vi "6733_Write_daqmx.vi"(0 "Arbitrary Waveform\nArray of Channels":T1(array[cluster])=[[{"AC Frequency (kHz)"=40.0, " Initial AC Ampl. (p-p/2)"=0.0, "Final AC Ampl."=0.0, "Initial DC Value"=-1.0, "Final DC Value"=-0.58, "Constant"=179.88, "Gamma AC"=1.0, "String"="Channel 0 A", "Gamma DC"=1.0}, {"AC Frequency (kHz)"=40.0, " Initial AC Ampl. (p-p/2)"=0.0, "Final AC Ampl."=0.0, "Initial DC Value"=-0.58, "Final DC Value"=-0.095, "Constant"=179.88, "Gamma AC"=1.0, "String"="Channel 0 B", "Gamma DC"=1.0}, {"AC Frequency (kHz)"=40.0, " Initial AC Ampl. (p-p/2)"=0.0, "Final AC Ampl."=0.0, "Initial DC Value"=-0.095, "Final DC Value"=-0.03, "Constant"=179.88, "Gamma AC"=1.0, "String"="Channel 0 C", "Gamma DC"=1.0}, {"AC Frequency (kHz)"=0.0, " Initial AC Ampl. (p-p/2)"=0.0, "Final AC Ampl."=0.0, "Initial DC Value"=0.0, "Final DC Value"=0.0, "Constant"=179.88, "Gamma AC"=0.0, "String"="Channel 0 D", "Gamma DC"=1.0}], [{"AC Frequency (kHz)"=10.0, " Initial AC Ampl. (p-p/2)"=5.0, "Final AC Ampl."=0.0, "Initial DC Value"=0.17, "Final DC Value"=0.095, "Constant"=0.25, "Gamma AC"=1.0, "String"="Channel 1 A", "Gamma DC"=1.0}, {"AC Frequency (kHz)"=10.0, " Initial AC Ampl. (p-p/2)"=5.0, "Final AC Ampl."=0.0, "Initial DC Value"=0.095, "Final DC Value"=0.009, "Constant"=0.25, "Gamma AC"=1.0, "String"="Channel 1 B", "Gamma DC"=1.0}, {"AC Frequency (kHz)"=10.0, " Initial AC Ampl. (p-p/2)"=0.0, "Final AC Ampl."=0.0, "Initial DC Value"=0.009, "Final DC Value"=0.001, "Constant"=0.25, "Gamma AC"=1.0, "String"="Channel 1 C", "Gamma DC"=1.0}, {"AC Frequency (kHz)"=0.0, " Initial AC Ampl. (p-p/2)"=0.0, "Final AC Ampl."=0.0, "Initial DC Value"=0.001, "Final DC Value"=0.001, "Constant"=0.25, "Gamma AC"=0.0, "String"="Channel 1 D", "Gamma DC"=1.0}], [{"AC Frequency (kHz)"=10.0, " Initial AC Ampl. (p-p/2)"=0.0, "Final AC Ampl."=0.0, "Initial DC Value"=0.006, "Final DC Value"=0.01, "Constant"=0.0, "Gamma AC"=1.0, "String"="Channel 2 A", "Gamma DC"=1.0}, {"AC Frequency (kHz)"=10.0, " Initial AC Ampl. (p-p/2)"=0.0, "Final AC Ampl."=0.0, "Initial DC Value"=0.01, "Final DC Value"=0.04, "Constant"=0.0, "Gamma AC"=1.0, "String"="Channel 2 B", "Gamma DC"=1.0}, {"AC Frequency (kHz)"=10.0, " Initial AC Ampl. (p-p/2)"=0.0, "Final AC Ampl."=0.0, "Initial DC Value"=0.04, "Final DC Value"=0.04, "Constant"=0.0, "Gamma AC"=1.0, "String"="Channel 2 C", "Gamma DC"=1.0}, {"AC Frequency (kHz)"=0.0, " Initial AC Ampl. (p-p/2)"=0.0, "Final AC Ampl."=0.0, "Initial DC Value"=0.04, "Final DC Value"=0.04, "Constant"=0.0, "Gamma AC"=0.0, "String"="Channel 2 D", "Gamma DC"=1.0}], [{"AC Frequency (kHz)"=10.0, " Initial AC Ampl. (p-p/2)"=0.0, "Final AC Ampl."=0.0, "Initial DC Value"=10.0, "Final DC Value"=10.0, "Constant"=199.2, "Gamma AC"=1.0, "String"="Channel 3 A", "Gamma DC"=1.0}, {"AC Frequency (kHz)"=10.0, " Initial AC Ampl. (p-p/2)"=0.0, "Final AC Ampl."=0.0, "Initial DC Value"=10.0, "Final DC Value"=1.0, "Constant"=199.2, "Gamma AC"=1.0, "String"="Channel 3 B", "Gamma DC"=1.0}, {"AC Frequency (kHz)"=10.0, " Initial AC Ampl. (p-p/2)"=0.0, "Final AC Ampl."=0.0, "Initial DC Value"=1.0, "Final DC Value"=0.9, "Constant"=199.2, "Gamma AC"=1.0, "String"="Channel 3 C", "Gamma DC"=1.0}, {"AC Frequency (kHz)"=0.0, " Initial AC Ampl. (p-p/2)"=0.0, "Final AC Ampl."=0.0, "Initial DC Value"=5.0, "Final DC Value"=5.0, "Constant"=199.2, "Gamma AC"=1.0, "String"="Channel 3 D", "Gamma DC"=1.0}], [{"AC Frequency (kHz)"=10.0, " Initial AC Ampl. (p-p/2)"=0.0, "Final AC Ampl."=0.0, "Initial DC Value"=2.445, "Final DC Value"=2.445, "Constant"=0.0, "Gamma AC"=1.0, "String"="Channel 4 A", "Gamma DC"=1.0}, {"AC Frequency (kHz)"=10.0, " Initial AC Ampl. (p-p/2)"=0.0, "Final AC Ampl."=0.0, "Initial DC Value"=2.445, "Final DC Value"=2.432, "Constant"=0.0, "Gamma AC"=1.0, "String"="Channel 4 B", "Gamma DC"=1.0}, {"AC Frequency (kHz)"=10.0, " Initial AC Ampl. (p-p/2)"=0.0, "Final AC Ampl."=0.0, "Initial DC Value"=2.432, "Final DC Value"=2.432, "Constant"=0.0, "Gamma AC"=1.0, "String"="Channel 4 C", "Gamma DC"=1.0}, {"AC Frequency (kHz)"=0.0, " Initial AC Ampl. (p-p/2)"=0.0, "Final AC Ampl."=0.0, "Initial DC Value"=2.432, "Final DC Value"=2.432, "Constant"=0.0, "Gamma AC"=0.0, "String"="Channel 4 D", "Gamma DC"=1.0}], [{"AC Frequency (kHz)"=10.0, " Initial AC Ampl. (p-p/2)"=0.0, "Final AC Ampl."=0.0, "Initial DC Value"=6.46, "Final DC Value"=6.46, "Constant"=0.0, "Gamma AC"=1.0, "String"="Channel 5 A", "Gamma DC"=1.0}, {"AC Frequency (kHz)"=10.0, " Initial AC Ampl. (p-p/2)"=0.0, "Final AC Ampl."=0.0, "Initial DC Value"=6.46, "Final DC Value"=6.46, "Constant"=0.0, "Gamma AC"=1.0, "String"="Channel 5 B", "Gamma DC"=1.0}, {"AC Frequency (kHz)"=10.0, " Initial AC Ampl. (p-p/2)"=0.0, "Final AC Ampl."=0.0, "Initial DC Value"=6.46, "Final DC Value"=6.46, "Constant"=0.0, "Gamma AC"=1.0, "String"="Channel 5 C", "Gamma DC"=1.0}, {"AC Frequency (kHz)"=0.0, " Initial AC Ampl. (p-p/2)"=0.0, "Final AC Ampl."=0.0, "Initial DC Value"=6.46, "Final DC Value"=6.46, "Constant"=0.0, "Gamma AC"=0.0, "String"="Channel 5 D", "Gamma DC"=1.0}], [{"AC Frequency (kHz)"=10.0, " Initial AC Ampl. (p-p/2)"=0.0, "Final AC Ampl."=0.0, "Initial DC Value"=6.98, "Final DC Value"=6.98, "Constant"=0.0, "Gamma AC"=1.0, "String"="Channel 6 A", "Gamma DC"=1.0}, {"AC Frequency (kHz)"=10.0, " Initial AC Ampl. (p-p/2)"=0.0, "Final AC Ampl."=0.0, "Initial DC Value"=6.98, "Final DC Value"=6.98, "Constant"=0.0, "Gamma AC"=1.0, "String"="Channel 6 B", "Gamma DC"=1.0}, {"AC Frequency (kHz)"=10.0, " Initial AC Ampl. (p-p/2)"=0.0, "Final AC Ampl."=0.0, "Initial DC Value"=6.98, "Final DC Value"=6.98, "Constant"=0.0, "Gamma AC"=1.0, "String"="Channel 6 C", "Gamma DC"=1.0}, {"AC Frequency (kHz)"=0.0, " Initial AC Ampl. (p-p/2)"=0.0, "Final AC Ampl."=0.0, "Initial DC Value"=6.98, "Final DC Value"=6.98, "Constant"=0.0, "Gamma AC"=0.0, "String"="Channel 6 D", "Gamma DC"=1.0}], [{"AC Frequency (kHz)"=10.0, " Initial AC Ampl. (p-p/2)"=0.0, "Final AC Ampl."=0.0, "Initial DC Value"=1.0, "Final DC Value"=1.0, "Constant"=0.0, "Gamma AC"=1.0, "String"="Channel 7 A", "Gamma DC"=1.0}, {"AC Frequency (kHz)"=10.0, " Initial AC Ampl. (p-p/2)"=0.0, "Final AC Ampl."=0.0, "Initial DC Value"=1.0, "Final DC Value"=1.0, "Constant"=0.0, "Gamma AC"=1.0, "String"="Channel 7 B", "Gamma DC"=1.0}, {"AC Frequency (kHz)"=10.0, " Initial AC Ampl. (p-p/2)"=0.0, "Final AC Ampl."=0.0, "Initial DC Value"=1.0, "Final DC Value"=1.0, "Constant"=0.0, "Gamma AC"=1.0, "String"="Channel 7 C", "Gamma DC"=1.0}, {"AC Frequency (kHz)"=0.0, " Initial AC Ampl. (p-p/2)"=0.0, "Final AC Ampl."=0.0, "Initial DC Value"=1.0, "Final DC Value"=1.0, "Constant"=0.0, "Gamma AC"=0.0, "String"="Channel 7 D", "Gamma DC"=1.0}]] {"Gamma DC" format="%.2f"; "Gamma AC" format="%.2f"; "Constant" min=0.0 max=240.0 format="%.2f"; "Final DC Value" format="%.3f"; "Initial DC Value" format="%.3f"; "Final AC Ampl." format="%.3f"; "Initial AC Ampl. (p-p/2)" format="%.3f"; "AC Frequency (kHz)" format="%.2f"}, 3 "Unit Conversions":u16[](array[ring])=[0, 1, 2, 3, 5, 2, 2, 2] items=["Freq (MHz) to Voltage 88Sr", "Dither Amplitude (% of max)", "B-field to Voltage", "Power Control V for 689 nm (%)", "Freq (MHz) to Voltage 86Sr", "Current (A) to Voltage Fet switch X trim"], 4 "Interval Lengths (ms)":dbl[](array[numeric])=[50.0, 150.0, 50.0, 50.0] format="%.3f", 5 "Channel Controls":bool[](array[boolean])=[TRUE, TRUE, TRUE, TRUE, TRUE, TRUE, TRUE, TRUE], 6 "ON or OFF?":bool[](array[boolean])=[TRUE, TRUE, TRUE, TRUE], 7 "Hold Final Value of Array?":bool=TRUE, 9 "error in":errorcluster, 12 "Dither Control":u16(ring)=1 items=["Disable Dither", "Enable Dither"]) -> (8 "Voltage\nArrays":dbl[][](graph), 10 "= Total Waveform\nTime (ms)":dbl=300.0 format="%.3f", 11 "Sampling\nRate":dbl=6788.9908256880735 format="%.2f", 14 "redMOTAOMVoltage":dbl=4.478911000000002, 15 "error out":errorcluster)   [LabVIEW 2013]
uses:
  <vilib>/Utility/error.llb/DialogType.ctl
  <vilib>/DAQmx/write.llb/DAQmx Write (Analog 1D Wfm NChan NSamp).vi
  <vilib>/DAQmx/configure/timing.llb/DAQmx Timing (Sample Clock).vi
  <vilib>/DAQmx/create/channels.llb/DAQmx Create Channel (CO-Pulse Generation-Frequency).vi
  <vilib>/DAQmx/configure/timing.llb/DAQmx Timing (Implicit).vi
  <vilib>/DAQmx/configure/trigger.llb/DAQmx Start Trigger (Digital Edge).vi
  Instance          13 24Saved   6733_Write_daqmx .vi
  <vilib>/DAQmx/miscellaneous.llb/DAQmx Fill In Error Info.vi
  <resource>/objmgr/daqmx.rc
panel:
  in  "Case Constant\n(See Context Help) 2":bool=TRUE
  in  "Dither Control":u16
  in  "Dither Control":u16
  in  "Case Constant\n(See Context Help)":bool
  in  "Dither Control":u16
  out "wvfrm size":i32=2036
  out "signal out":waveform(dbl)[](graph)=[{"t0"=timestamp(0 s since 1904-01-01), "dt"=0.0001472972972972973, "Y"=array[2036 elements]}, {"t0"=timestamp(0 s since 1904-01-01), "dt"=0.0001472972972972973, "Y"=array[2036 elements]}, {"t0"=timestamp(0 s since 1904-01-01), "dt"=0.0001472972972972973, "Y"=array[2036 elements]}, {"t0"=timestamp(0 s since 1904-01-01), "dt"=0.0001472972972972973, "Y"=array[2036 elements]}, {"t0"=timestamp(0 s since 1904-01-01), "dt"=0.0001472972972972973, "Y"=array[2036 elements]}, {"t0"=timestamp(0 s since 1904-01-01), "dt"=0.0001472972972972973, "Y"=array[2036 elements]}, {"t0"=timestamp(0 s since 1904-01-01), "dt"=0.0001472972972972973, "Y"=array[2036 elements]}, {"t0"=timestamp(0 s since 1904-01-01), "dt"=0.0001472972972972973, "Y"=array[2036 elements]}]
  out "6733 counter task out":refnum<k21>="6733 Counter Output"
  out "6733 adiabatic loading task out":refnum<k21>="Red Waveform"
  out "6733 Status":string="PCI-6733 OK"
  out "total points\nper channel":dbl=2036.0 format="%.2f"
  out "Points per Segment":dbl[](array[numeric])=[339.0, 1018.0, 339.0, 339.0] format="%.2f"
  # "Controls"
  # "Warning! Constant for interval A does not set all intervals for 86 Sr frequency"
  # "Note: B-field to Voltage\nConversion not yet\nimplemented.  Must \ninsert appropriate\nformulae."
  # "Don't change"
  # "Interval A"
  # "Interval B"
  # "Interval C"
  # "Interval D"
  # "Output"
  # "Must use all channels"
  # "CH 0"
  # "CH 1"
  # "CH 2"
  # "CH 3"
  # "CH 4"
  # "CH 5"
  # "CH 6"
  # "CH 7"
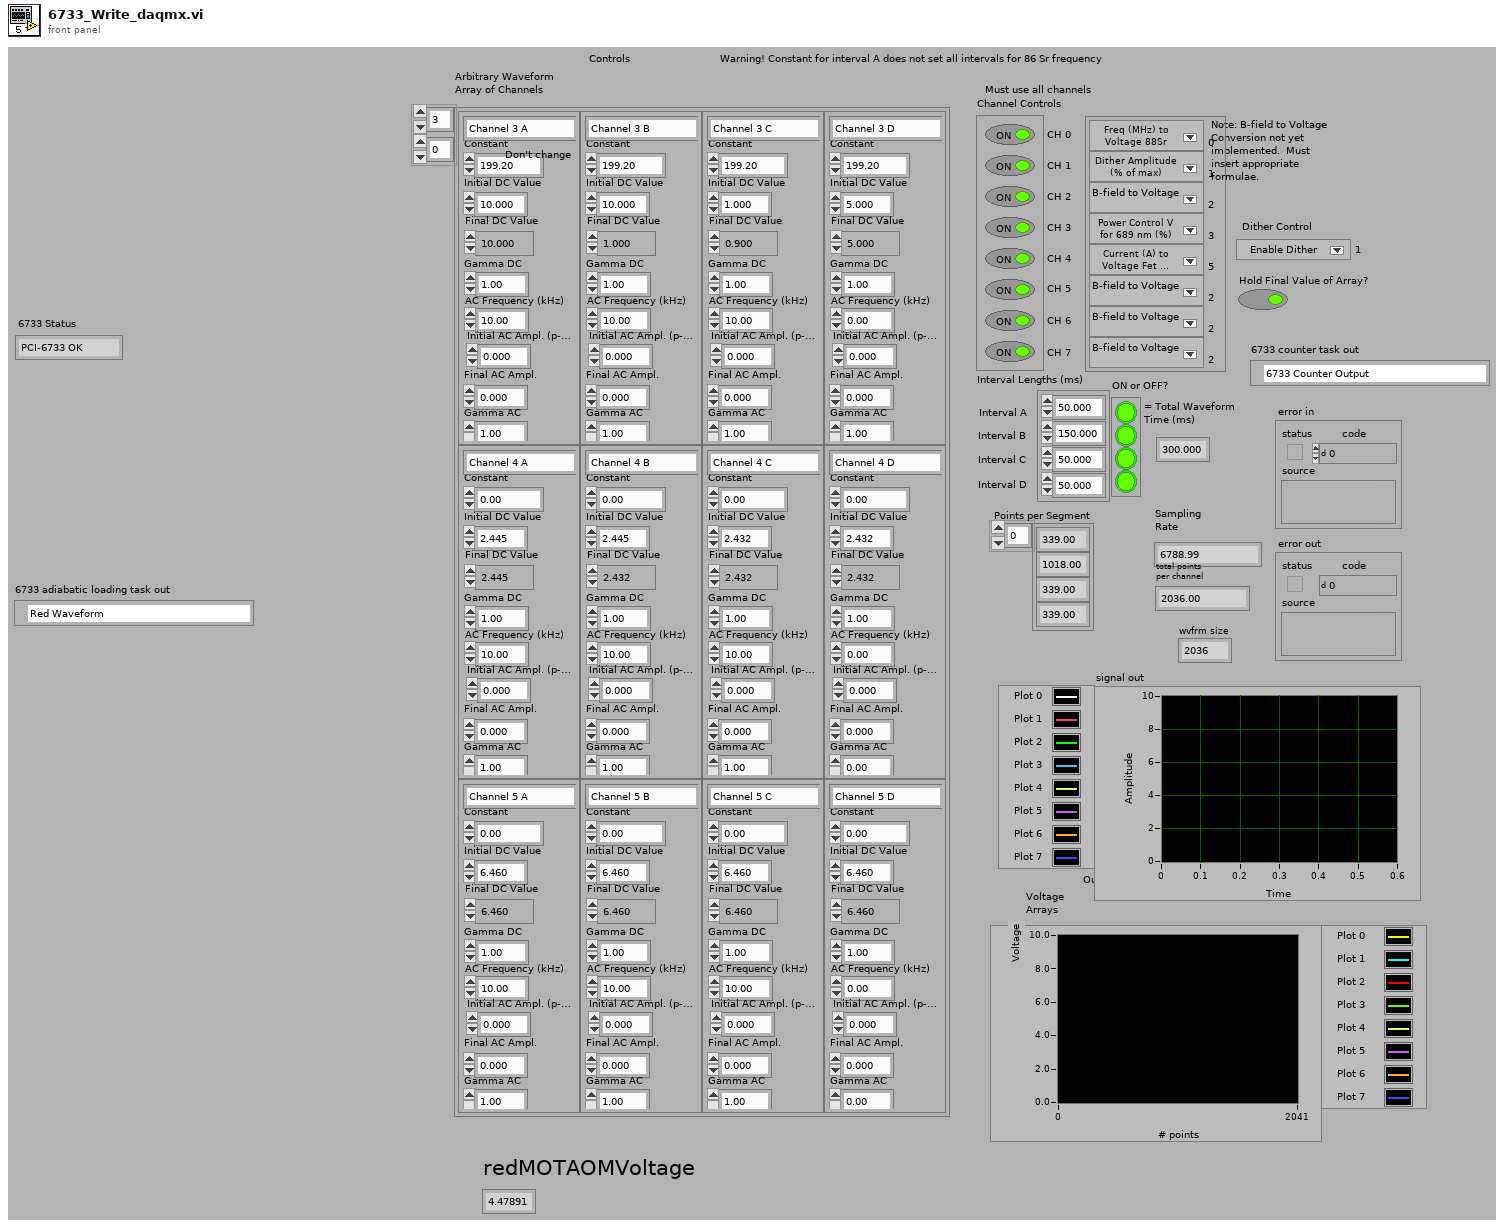
[diagram p1: front panel]
types:
  T1 = cluster{"AC Frequency (kHz)":dbl, " Initial AC Ampl. (p-p/2)":dbl, "Final AC Ampl.":dbl, "Initial DC Value":dbl, "Final DC Value":dbl, "Constant":dbl, "Gamma AC":dbl, "String":string, "Gamma DC":dbl}[][]
  T2 = cluster{"AC Frequency (kHz)":dbl, " Initial AC Ampl. (p-p/2)":dbl, "Final AC Ampl.":dbl, "Initial DC Value":dbl, "Final DC Value":dbl, "Constant":dbl, "Gamma AC":dbl, "String":string, "Gamma DC":dbl}
  T3 = typedef "DialogType.ctl" = u16
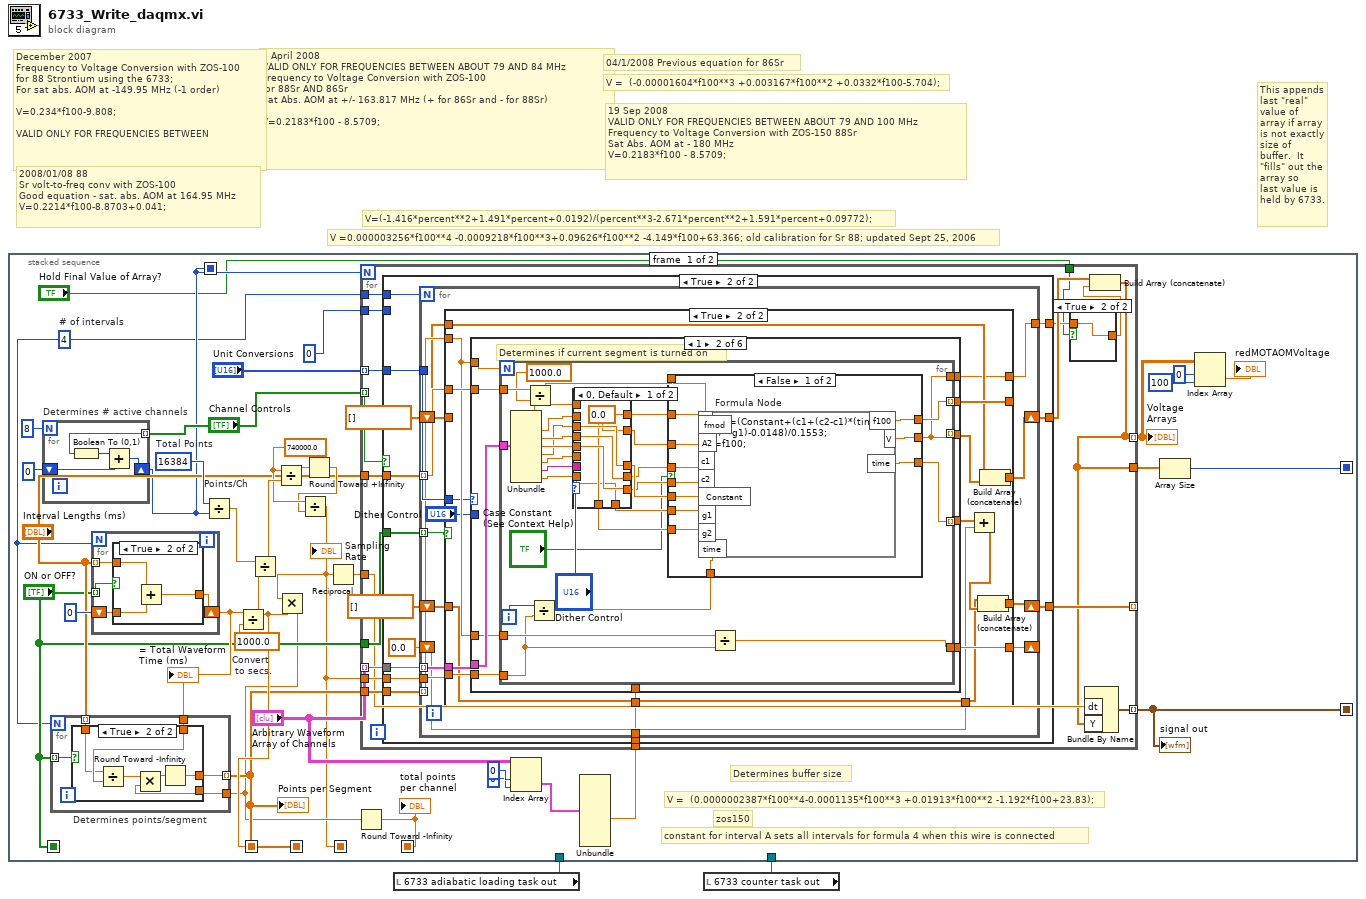
[diagram p0: block diagram]
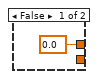
[diagram p2: hidden frame]
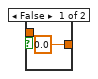
[diagram p4: hidden frame]
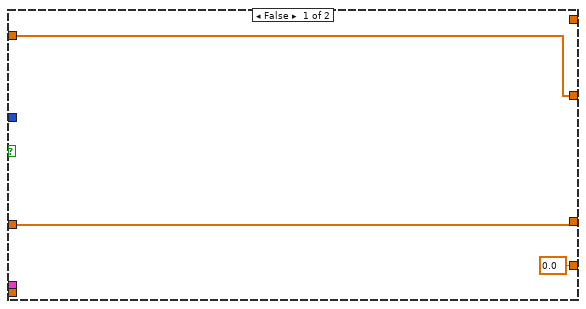
[diagram p6: hidden frame]
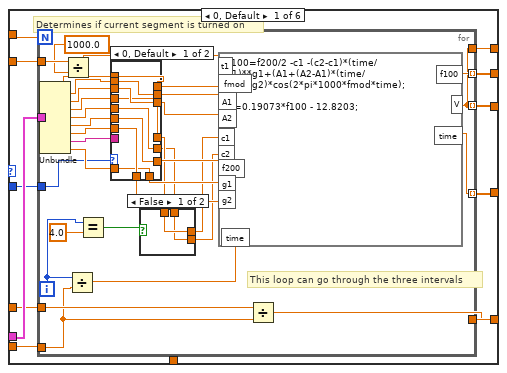
[diagram p7: hidden frame]
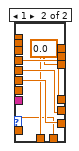
[diagram p9: hidden frame]
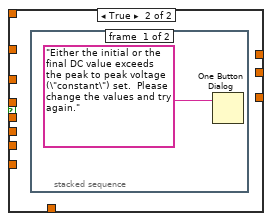
[diagram p10: hidden frame]
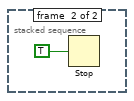
[diagram p11: hidden frame]
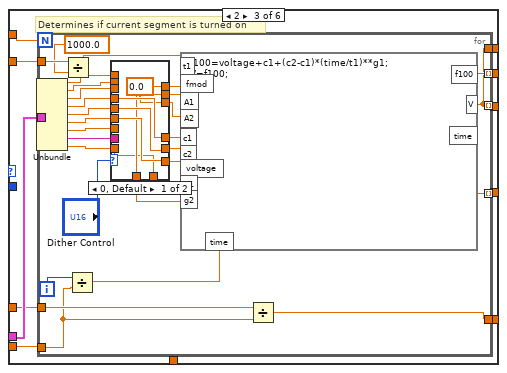
[diagram p13: hidden frame]
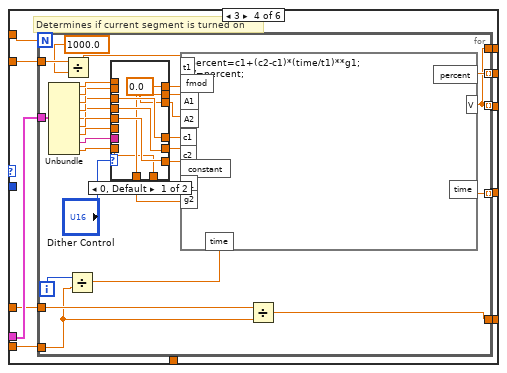
[diagram p15: hidden frame]
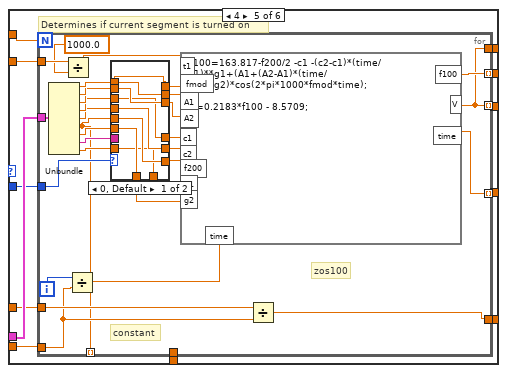
[diagram p17: hidden frame]
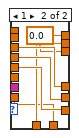
[diagram p18: hidden frame]
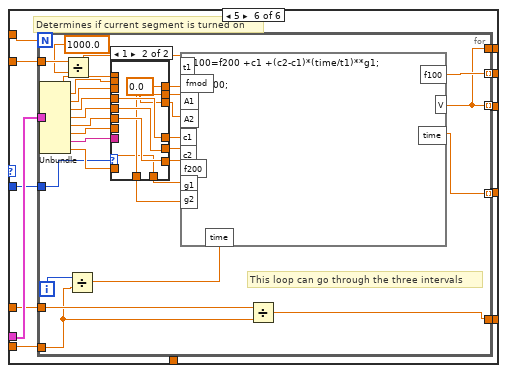
[diagram p19: hidden frame]
diagram:
  # "19 Sep 2008\nVALID ONLY FOR FREQUENCIES BETWEEN ABOUT 79 AND 100 MHz\nFrequency to Voltage Conversion with ZOS-150 88Sr\nSat Abs. AOM at - 180 MHz\nV=0.2183*f100 - 8.5709;"
  # "7 April 2008\nVALID ONLY FOR FREQUENCIES BETWEEN ABOUT 79 AND 84 MHz\nFrequency to Voltage Conversion with ZOS-100\nfor 88Sr AND 86Sr\nSat Abs. AOM at +/- 163.817 MHz (+ for 86Sr and - for 88Sr)\n\nV=0.2183*f100 - 8.5709;"
  # "04/1/2008 Previous equation for 86Sr"
  # "V =  (-0.00001604*f100**3 +0.003167*f100**2 +0.0332*f100-5.704);"
  # "December 2007\nFrequency to Voltage Conversion with ZOS-100\nfor 88 Strontium using the 6733; \nFor sat abs. AOM at -149.95 MHz (-1 order)\n\nV=0.234*f100-9.808;\n\nVALID ONLY FOR FREQUENCIES BETWEEN"
  # "2008/01/08 88\nSr volt-to-freq conv with ZOS-100\nGood equation - sat. abs. AOM at 164.95 MHz\nV=0.2214*f100-8.8703+0.041;"
  # "This appends\nlast \"real\"\nvalue of\narray if array \nis not exactly\nsize of \nbuffer.  It\n\"fills\" out the\narray so \nlast value is\nheld by 6733."
  # "V =0.000003256*f100**4 -0.0009218*f100**3+0.09626*f100**2 -4.149*f100+63.366; old calibration for Sr 88; updated Sept 25, 2006"
  # "V=(-1.416*percent**2+1.491*percent+0.0192)/(percent**3-2.671*percent**2+1.591*percent+0.09772);"
  n1 = local read "6733 adiabatic loading task out"() -> (w2:refnum<k21>)
  n2 = local read "6733 counter task out"() -> (w1:refnum<k21>)
  n3 = stacked-sequence {
    seq-local: [w10 _] -> [_ w476]
    seq-local: [w23 _] -> [_ _]
    seq-local: ["ON or OFF?" _] -> [_ _]
    seq-local: [w20 _] -> [_ _]
    seq-local: [w25 _] -> [_ _]
    seq-local: [w14 _] -> [_ w523]
    seq-local: [w11 _] -> [_ w475]
    seq-local: [w8 _] -> [_ w474]
    tunnel: w2 -> [_ w514]
    tunnel: w1 -> [_ w513]
    frame #0 {
      w29 = 740000.0 ("x")
      w7 = 4  # # of intervals
      w39 = 16384  # Total Points
      # "zos150"
      # "Determines buffer size"
      # "constant for interval A sets all intervals for formula 4 when this wire is connected"
      # "V =  (0.0000002387*f100**4-0.0001135*f100**3 +0.01913*f100**2 -1.192*f100+23.83);"
      n4 = for "Determines # active channels" {
        N: 8 -> [_]
        tunnel: "Channel Controls" -> [w63] mode=indexing
        shift-right: [w60] -> w14
        shift-left: 0 -> [w61]
        n5 = Boolean To (0,1)(Boolean=w63) -> (0, 1=w62:i16)
        n6 = Add(x=w62, y=w61) -> (x+y=w60:i32)
      }
      n7 = for {
        N: w7 -> [_]
        tunnel: "Interval Lengths (ms)" -> [w53] mode=indexing
        tunnel: "ON or OFF?" -> [w55] mode=indexing
        shift-right: [w52] -> w26
        shift-left: 0 -> [w54]
        n8 = case shown="True" w55 {
          tunnel: w54 -> [w56 w59]
          tunnel: w53 -> [_ w58]
          tunnel: [w56 w57] -> w52
          frame False {
          }
          frame True {
            n9 = Add(x=w58, y=w59) -> (x+y=w57:dbl)
          }
        }
      }
      "= Total Waveform\nTime (ms)" <- w26
      n10 = Divide "Points/Ch"(x=w39, y=w14) -> (x/y=w24:dbl)
      n11 = Divide "Convert\n to secs."(x=w26, y=1000.0) -> (x/y=w25:dbl)
      n12 = Divide(x=w24, y=w25) -> (x/y=w31:dbl)
      n13 = Divide(x=w29, y=w31) -> (x/y=w30:dbl)
      n14 = Round Toward +Infinity(x=w30) -> (ceil(x): smallest int >= x=w28:dbl)
      n15 = Divide(x=w29, y=w28) -> (x/y=w10:dbl)
      "Sampling\nRate" <- w10
      n16 = Multiply(x=w10, y=w25) -> (x*y=w21:dbl)
      n17 = for "Determines points/segment" {
        N: w7 -> [_]
        tunnel: "ON or OFF?" -> [w44] mode=indexing
        tunnel: "Interval Lengths (ms)" -> [w43] mode=indexing
        tunnel: w26 -> [w42]
        tunnel: [w41] -> w23 mode=indexing
        tunnel: w21 -> [w40]
        n18 = case shown="True" w44 {
          tunnel: w43 -> [_ w50]
          tunnel: w42 -> [_ w51]
          tunnel: [0.0 w47] -> w41
          tunnel: w40 -> [_ w48]
          frame False {
          }
          frame True {
            n19 = Divide(x=w50, y=w51) -> (x/y=w49:dbl)
            n20 = Multiply(x=w49, y=w48) -> (x*y=w46:dbl)
            n21 = Round Toward -Infinity(1:w46) -> (0:w47:dbl)
          }
        }
      }
      "Points per Segment" <- w23
      n22 = Reciprocal(x=w10) -> (1/x=w12:dbl)
      n23 = Round Toward -Infinity(1:w21) -> (0:w20:dbl)
      "total points\nper channel" <- w20
      n24 = Index Array(array="Arbitrary Waveform\nArray of Channels", index (row)=0, index (col)=0 ("disabled index (col)")) -> (element=w16:T2)
      n25 = Unbundle(w16) -> ("Constant"=w15:dbl)  [unwired: 8 out]
      n26 = for {
        N: w14 -> [_]
        tunnel: "Channel Controls" -> [w81] mode=indexing
        tunnel: 0 -> [w80]
        tunnel: "Unit Conversions" -> [w78] mode=indexing
        tunnel: "Arbitrary Waveform\nArray of Channels" -> [w79] mode=indexing
        tunnel: w23 -> [w77]
        tunnel: w10 -> [w67]
        tunnel: "Interval Lengths (ms)" -> [w76]
        tunnel: "ON or OFF?" -> [w75]
        tunnel: [w74] -> _ mode=indexing
        tunnel: [w64] -> w6 mode=indexing
        tunnel: w15 -> [w73]
        tunnel: "Hold Final Value of Array?" -> [w69]
        tunnel: [w68] -> w11 mode=indexing
        tunnel: w12 -> [w66]
        tunnel: [w64] -> w9
        tunnel: w7 -> [w65]
        n27 = case shown="True" w81 {
          tunnel: w80 -> [_ _]
          tunnel: w79 -> [_ w97]
          tunnel: w78 -> [_ w96]
          tunnel: w77 -> [_ w95]
          tunnel: w67 -> [_ w94]
          tunnel: w76 -> [_ w93]
          tunnel: w75 -> [_ w92]
          tunnel: [_ w90] -> w74
          tunnel: [_ w88] -> w72
          tunnel: w73 -> [_ w86]
          tunnel: [_ w85] -> w71
          tunnel: w65 -> [_ w84]
          frame False {
          }
          frame True {
            n28 = for {
              N: w84 -> [_]
              tunnel: w97 -> [w109] mode=indexing
              tunnel: w96 -> [w111]
              tunnel: w95 -> [w110] mode=indexing
              tunnel: w94 -> [w108]
              tunnel: w93 -> [w107] mode=indexing
              tunnel: w92 -> [w106] mode=indexing
              shift-right: [w105] -> w90
              shift-left: dbl[] [] -> [w104]
              shift-right: [w103] -> _
              shift-left: 0.0 -> [w102]
              shift-right: [w101] -> w88
              shift-left: dbl[] [] -> [w100]
              tunnel: w86 -> [w99]
              tunnel: [w98] -> w85
              n29 = case shown="True" w106 {
                tunnel: w111 -> [_ w118]
                tunnel: w110 -> [_ w124]
                tunnel: w109 -> [_ w132]
                tunnel: w108 -> [_ w131]
                tunnel: w107 -> [_ w130]
                tunnel: [_ w129] -> _
                tunnel: [w114 w128] -> w105
                tunnel: w104 -> [w114 w122]
                tunnel: [0.0 w126] -> w103
                tunnel: w102 -> [_ w125]
                tunnel: [w112 w121] -> w101
                tunnel: w100 -> [_ w119]
                tunnel: w100 -> [w112 _]
                tunnel: w99 -> [_ w116]
                tunnel: [_ w115] -> w98
                frame False {
                }
                frame True {
                  n30 = case shown="1" w118 {
                    tunnel: w124 -> [w143 w203 w268 w321 w376 w430]
                    tunnel: w132 -> [w142 w202 w267 w320 w375 w429]
                    tunnel: w131 -> [w137 w197 w262 w315 w370 w424]
                    tunnel: w130 -> [w141 w201 w266 w319 w374 w428]
                    tunnel: [w140 w200 w265 w318 w373 w427] -> w129
                    tunnel: [w139 w199 w264 w317 w372 w426] -> w120
                    tunnel: [w138 w198 w263 w316 w371 w425] -> w127
                    tunnel: [w136 w196 w261 w314 w369 w423] -> w126
                    tunnel: w124 -> [w135 w195 w260 w313 w368 w422]
                    tunnel: "Dither Control" -> [w134 _ _ _ w367 w421]
                    tunnel: w116 -> [_ _ _ _ w366 _]
                    tunnel: [w133 w194 w259 w312 w365 w420] -> w115
                    frame 0, Default {
                      # "Determines if current segment is turned on"
                      n31 = for {
                        N: w143 -> [_]
                        tunnel: w142 -> [w177]
                        tunnel: w137 -> [w158]
                        tunnel: w141 -> [w176]
                        tunnel: [w152] -> w139 mode=indexing
                        tunnel: [w156] -> w138 mode=indexing
                        tunnel: [w155] -> w140 mode=indexing
                        tunnel: [w157] -> w136
                        tunnel: w135 -> [w159]
                        tunnel: w134 -> [w154]
                        tunnel: [w152] -> w133
                        i -> [w145]
                        # "EQUATION TO USE WITH SAT. ABS. AOM AT -180 MHz FOR 88SR:\nV=0.19073*f100 - 12.8203"
                        # "This loop can go through the three intervals"
                        n32 = Unbundle(w177) -> ("AC Frequency (kHz)"=w171:dbl, "Initial AC Ampl. (p-p/2)"=w170:dbl, "Final AC Ampl."=w169:dbl, "Initial DC Value"=w153:dbl, "Final DC Value"=w168:dbl, "Constant"=w172:dbl, "Gamma AC"=w173:dbl, "String"=w174:string, "Gamma DC"=w162:dbl)
                        n33 = Divide(x=w176, y=1000.0) -> (x/y=w144:dbl)
                        n34 = Divide(x=w145, y=w158) -> (x/y=w160:dbl)
                        n35 = Equal?(x=w145, y=4.0) -> (x = y?=w150:bool)
                        n36 = case shown="0, Default" w154 {
                          tunnel: w174 -> [_ _]
                          tunnel: w173 -> [w182 _]
                          tunnel: w172 -> [w183 w191]
                          tunnel: w171 -> [w188 _]
                          tunnel: w170 -> [w187 _]
                          tunnel: w169 -> [w186 _]
                          tunnel: w153 -> [w185 w193]
                          tunnel: w168 -> [w184 w192]
                          tunnel: [w188 w190] -> w167
                          tunnel: [w187 w190] -> w166
                          tunnel: [w186 w190] -> w165
                          tunnel: [w185 w193] -> w149
                          tunnel: [w184 w192] -> w148
                          tunnel: [w183 w191] -> w164
                          tunnel: [w182 w190] -> w163
                          tunnel: w162 -> [w181 w189]
                          tunnel: [w181 w189] -> w161
                          frame 0, Default {
                          }
                          frame 1 {
                            w190 = 0.0 ("AC Frequency (kHz)")
                          }
                        }
                        n37 = case shown="False" w150 {
                          tunnel: [w179 w180] -> w147
                          tunnel: w149 -> [w179 w180]
                          tunnel: [w178 w180] -> w146
                          tunnel: w148 -> [w178 _]
                          frame False {
                          }
                          frame True {
                          }
                        }
                        n38 = formula code="f100=f200/2 -c1 -(c2-c1)*(time/t1)**g1+(A1+(A2-A1)*(time/t1)**g2)*cos(2*pi*1000*fmod*time);\n\nV=0.19073*f100 - 12.8203;"("c1"=w147, "time"=w160, "t1"=w144, "c2"=w146, "f200"=w164, "fmod"=w167, "A1"=w166, "A2"=w165, "g1"=w161, "g2"=w163) -> ("f100"=w155:dbl, "time"=w156:dbl, "V"=w152:dbl)
                        n39 = Divide(x=w159, y=w158) -> (x/y=w157:dbl)
                      }
                    }
                    frame 1 {
                      # "Determines if current segment is turned on"
                      n40 = for {
                        N: w203 -> [_]
                        tunnel: w202 -> [w232]
                        tunnel: w197 -> [w216]
                        tunnel: w201 -> [w229]
                        tunnel: [w205] -> w199 mode=indexing
                        tunnel: [w231] -> w198 mode=indexing
                        tunnel: [w230] -> w200 mode=indexing
                        tunnel: [w215] -> w196
                        tunnel: w195 -> [w217]
                        tunnel: [w205] -> w194
                        i -> [w227]
                        n41 = Unbundle(w232) -> ("AC Frequency (kHz)"=w209:dbl, "Final AC Ampl."=w210:dbl, "Initial DC Value"=w213:dbl, "Final DC Value"=w212:dbl, "Constant"=w211:dbl, "Gamma AC"=w225:dbl, "String"=w226:string, "Gamma DC"=w220:dbl)  [unwired: 1 out]
                        n42 = Divide(x=w229, y=1000.0) -> (x/y=w224:dbl)
                        n43 = Divide(x=w227, y=w216) -> (x/y=w218:dbl)
                        n44 = case shown="0, Default" "Dither Control" {
                          tunnel: w226 -> [_ _]
                          tunnel: w225 -> [_ w254]
                          tunnel: w212 -> [w249 w255]
                          tunnel: w210 -> [_ w258]
                          tunnel: w211 -> [w251 w257]
                          tunnel: w213 -> [w250 w256]
                          tunnel: [w248 w252] -> w223
                          tunnel: [w248 w258] -> w222
                          tunnel: [w251 w257] -> w208
                          tunnel: [w250 w256] -> w207
                          tunnel: [w249 w255] -> w206
                          tunnel: [w248 w254] -> w221
                          tunnel: w220 -> [w247 w253]
                          tunnel: [w247 w253] -> w219
                          tunnel: w209 -> [_ w252]
                          frame 0, Default {
                            w248 = 0.0 ("AC Frequency (kHz)")
                          }
                          frame 1 {
                          }
                        }
                        n45 = case shown="False" "Case Constant\n(See Context Help)" {
                          tunnel: [w244 _] -> w205
                          tunnel: [w243 _] -> w231
                          tunnel: [w242 _] -> w230
                          tunnel: w224 -> [w241 _]
                          tunnel: w223 -> [w240 _]
                          tunnel: w222 -> [w239 _]
                          tunnel: w221 -> [w238 _]
                          tunnel: w219 -> [w237 _]
                          tunnel: w218 -> [w236 _]
                          tunnel: w207 -> [w235 _]
                          tunnel: w206 -> [w234 _]
                          tunnel: w208 -> [w233 _]
                          frame False {
                            # "Dither amplitude control"
                            n46 = formula code="f100=(Constant+(c1+(c2-c1)*(time/t1)**g1)-0.0148)/0.1553;\nV=f100;"("c1"=w235, "time"=w236, "t1"=w241, "c2"=w234, "Constant"=w233, "fmod"=w240, "A2"=w239, "g1"=w237, "g2"=w238) -> ("f100"=w242:dbl, "time"=w243:dbl, "V"=w244:dbl)
                          }
                          frame True {
                            n47 = stacked-sequence {
                              frame #0 {
                                n48 = One Button Dialog(message="Either the initial or the final DC value exceeds the peak to peak voltage (\"constant\") set.  Please change the values and try again.") -> ()  [unwired: 1 in, 1 out]
                              }
                              frame #1 {
                                n49 = Stop(stop? (T)=TRUE) -> ()
                              }
                            }
                          }
                        }
                        n50 = Divide(x=w217, y=w216) -> (x/y=w215:dbl)
                      }
                    }
                    frame 2 {
                      # "Determines if current segment is turned on"
                      n51 = for {
                        N: w268 -> [_]
                        tunnel: w267 -> [w298]
                        tunnel: w262 -> [w272]
                        tunnel: w266 -> [w295]
                        tunnel: [w269] -> w264 mode=indexing
                        tunnel: [w297] -> w263 mode=indexing
                        tunnel: [w296] -> w265 mode=indexing
                        tunnel: [w271] -> w261
                        tunnel: w260 -> [w273]
                        tunnel: [w269] -> w259
                        i -> [w293]
                        # "B-field to voltage"
                        n52 = Unbundle(w298) -> ("AC Frequency (kHz)"=w289:dbl, "Initial AC Ampl. (p-p/2)"=w288:dbl, "Final AC Ampl."=w287:dbl, "Initial DC Value"=w286:dbl, "Final DC Value"=w285:dbl, "Constant"=w290:dbl, "Gamma AC"=w291:dbl, "String"=w292:string, "Gamma DC"=w276:dbl)
                        n53 = Divide(x=w295, y=1000.0) -> (x/y=w284:dbl)
                        n54 = Divide(x=w293, y=w272) -> (x/y=w274:dbl)
                        n55 = case shown="0, Default" "Dither Control" {
                          tunnel: w292 -> [_ _]
                          tunnel: w291 -> [_ w305]
                          tunnel: w290 -> [w301 w306]
                          tunnel: w289 -> [_ w311]
                          tunnel: w288 -> [_ w310]
                          tunnel: w287 -> [_ w309]
                          tunnel: w286 -> [w303 w308]
                          tunnel: w285 -> [w302 w307]
                          tunnel: [w300 w311] -> w283
                          tunnel: [w300 w310] -> w282
                          tunnel: [w300 w309] -> w281
                          tunnel: [w303 w308] -> w280
                          tunnel: [w302 w307] -> w279
                          tunnel: [w301 w306] -> w278
                          tunnel: [w300 w305] -> w277
                          tunnel: w276 -> [w299 w304]
                          tunnel: [w299 w304] -> w275
                          frame 0, Default {
                            w300 = 0.0 ("AC Frequency (kHz)")
                          }
                          frame 1 {
                          }
                        }
                        n56 = formula code="f100=voltage+c1+(c2-c1)*(time/t1)**g1;\nV=f100;"("c1"=w280, "time"=w274, "t1"=w284, "c2"=w279, "voltage"=w278, "fmod"=w283, "A1"=w282, "A2"=w281, "g1"=w275, "g2"=w277) -> ("f100"=w296:dbl, "time"=w297:dbl, "V"=w269:dbl)
                        n57 = Divide(x=w273, y=w272) -> (x/y=w271:dbl)
                      }
                    }
                    frame 3 {
                      # "Determines if current segment is turned on"
                      n58 = for {
                        N: w321 -> [_]
                        tunnel: w320 -> [w351]
                        tunnel: w315 -> [w325]
                        tunnel: w319 -> [w348]
                        tunnel: [w322] -> w317 mode=indexing
                        tunnel: [w350] -> w316 mode=indexing
                        tunnel: [w349] -> w318 mode=indexing
                        tunnel: [w324] -> w314
                        tunnel: w313 -> [w326]
                        tunnel: [w322] -> w312
                        i -> [w346]
                        # "Power Control Voltage for 689 nm\npercent = 1 is full power"
                        n59 = Unbundle(w351) -> ("AC Frequency (kHz)"=w342:dbl, "Initial AC Ampl. (p-p/2)"=w341:dbl, "Final AC Ampl."=w340:dbl, "Initial DC Value"=w339:dbl, "Final DC Value"=w338:dbl, "Constant"=w343:dbl, "Gamma AC"=w344:dbl, "String"=w345:string, "Gamma DC"=w329:dbl)
                        n60 = Divide(x=w348, y=1000.0) -> (x/y=w337:dbl)
                        n61 = Divide(x=w346, y=w325) -> (x/y=w327:dbl)
                        n62 = case shown="0, Default" "Dither Control" {
                          tunnel: w345 -> [_ _]
                          tunnel: w344 -> [_ w358]
                          tunnel: w343 -> [w354 w359]
                          tunnel: w342 -> [_ w364]
                          tunnel: w341 -> [_ w363]
                          tunnel: w340 -> [_ w362]
                          tunnel: w339 -> [w356 w361]
                          tunnel: w338 -> [w355 w360]
                          tunnel: [w353 w364] -> w336
                          tunnel: [w353 w363] -> w335
                          tunnel: [w353 w362] -> w334
                          tunnel: [w356 w361] -> w333
                          tunnel: [w355 w360] -> w332
                          tunnel: [w354 w359] -> w331
                          tunnel: [w353 w358] -> w330
                          tunnel: w329 -> [w352 w357]
                          tunnel: [w352 w357] -> w328
                          frame 0, Default {
                            w353 = 0.0 ("AC Frequency (kHz)")
                          }
                          frame 1 {
                          }
                        }
                        n63 = formula code="percent=c1+(c2-c1)*(time/t1)**g1;\nV=percent;"("c1"=w333, "time"=w327, "t1"=w337, "c2"=w332, "constant"=w331, "fmod"=w336, "A1"=w335, "A2"=w334, "g1"=w328, "g2"=w330) -> ("percent"=w349:dbl, "time"=w350:dbl, "V"=w322:dbl)
                        n64 = Divide(x=w326, y=w325) -> (x/y=w324:dbl)
                      }
                    }
                    frame 4 {
                      # "Determines if current segment is turned on"
                      n65 = for {
                        N: w376 -> [_]
                        tunnel: w375 -> [w406]
                        tunnel: w370 -> [w383]
                        tunnel: w374 -> [w405]
                        tunnel: [w377] -> w372 mode=indexing
                        tunnel: [w381] -> w371 mode=indexing
                        tunnel: [w380] -> w373 mode=indexing
                        tunnel: [w382] -> w369
                        tunnel: w368 -> [w384]
                        tunnel: w367 -> [w379]
                        tunnel: w366 -> [_]
                        tunnel: [w378] -> _ mode=indexing
                        tunnel: [w377] -> w365
                        i -> [w403]
                        # "zos100"
                        # "Frequency to Voltage Conversion for 6733\nwith 86 Strontium zos100\nSat Abs. AOM at 163.817 MHz (+1 order)\n\nUPDATED 01 APRIL 2008"
                        # "constant"
                        n66 = Unbundle(w406) -> ("AC Frequency (kHz)"=w400:dbl, "Initial AC Ampl. (p-p/2)"=w399:dbl, "Final AC Ampl."=w398:dbl, "Initial DC Value"=w397:dbl, "Final DC Value"=w396:dbl, "Constant"=w378:dbl, "Gamma AC"=w401:dbl, "String"=w402:string, "Gamma DC"=w387:dbl)
                        n67 = Divide(x=w405, y=1000.0) -> (x/y=w395:dbl)
                        n68 = Divide(x=w403, y=w383) -> (x/y=w385:dbl)
                        n69 = case shown="0, Default" w379 {
                          tunnel: w402 -> [_ _]
                          tunnel: w401 -> [w408 _]
                          tunnel: w378 -> [w409 w417]
                          tunnel: w400 -> [w414 _]
                          tunnel: w399 -> [w413 _]
                          tunnel: w398 -> [w412 _]
                          tunnel: w397 -> [w411 w419]
                          tunnel: w396 -> [w410 w418]
                          tunnel: [w414 w416] -> w394
                          tunnel: [w413 w416] -> w393
                          tunnel: [w412 w416] -> w392
                          tunnel: [w411 w419] -> w391
                          tunnel: [w410 w418] -> w390
                          tunnel: [w409 w417] -> w389
                          tunnel: [w408 w416] -> w388
                          tunnel: w387 -> [w407 w415]
                          tunnel: [w407 w415] -> w386
                          frame 0, Default {
                          }
                          frame 1 {
                            w416 = 0.0 ("AC Frequency (kHz)")
                          }
                        }
                        n70 = formula code="f100=163.817-f200/2 -c1 -(c2-c1)*(time/t1)**g1+(A1+(A2-A1)*(time/t1)**g2)*cos(2*pi*1000*fmod*time);\n\nV=0.2183*f100 - 8.5709;"("c1"=w391, "time"=w385, "t1"=w395, "c2"=w390, "f200"=w389, "fmod"=w394, "A1"=w393, "A2"=w392, "g1"=w386, "g2"=w388) -> ("f100"=w380:dbl, "time"=w381:dbl, "V"=w377:dbl)
                        n71 = Divide(x=w384, y=w383) -> (x/y=w382:dbl)
                      }
                    }
                    frame 5 {
                      # "Determines if current segment is turned on"
                      n72 = for {
                        N: w430 -> [_]
                        tunnel: w429 -> [w460]
                        tunnel: w424 -> [w437]
                        tunnel: w428 -> [w459]
                        tunnel: [w431] -> w426 mode=indexing
                        tunnel: [w435] -> w425 mode=indexing
                        tunnel: [w434] -> w427 mode=indexing
                        tunnel: [w436] -> w423
                        tunnel: w422 -> [w438]
                        tunnel: w421 -> [w433]
                        tunnel: [w431] -> w420
                        i -> [w457]
                        # "Use V=c1 to be able to change c1 and c2\nprovided c1 and c2 match."
                        # "current to voltage conversion for FET\n switch  driving X trim coils. Derivation on\n Neutrals Notebook A pg 87 yellow"
                        # "This loop can go through the three intervals"
                        n73 = Unbundle(w460) -> ("AC Frequency (kHz)"=w453:dbl, "Initial AC Ampl. (p-p/2)"=w452:dbl, "Final AC Ampl."=w451:dbl, "Initial DC Value"=w432:dbl, "Final DC Value"=w450:dbl, "Constant"=w454:dbl, "Gamma AC"=w455:dbl, "String"=w456:string, "Gamma DC"=w441:dbl)
                        n74 = Divide(x=w459, y=1000.0) -> (x/y=w449:dbl)
                        n75 = Divide(x=w457, y=w437) -> (x/y=w439:dbl)
                        n76 = case shown="1" w433 {
                          tunnel: w456 -> [_ _]
                          tunnel: w455 -> [w462 _]
                          tunnel: w454 -> [w463 w471]
                          tunnel: w453 -> [w468 _]
                          tunnel: w452 -> [w467 _]
                          tunnel: w451 -> [w466 _]
                          tunnel: w432 -> [w465 w473]
                          tunnel: w450 -> [w464 w472]
                          tunnel: [w468 w470] -> w448
                          tunnel: [w467 w470] -> w447
                          tunnel: [w466 w470] -> w446
                          tunnel: [w465 w473] -> w445
                          tunnel: [w464 w472] -> w444
                          tunnel: [w463 w471] -> w443
                          tunnel: [w462 w470] -> w442
                          tunnel: w441 -> [w461 w469]
                          tunnel: [w461 w469] -> w440
                          frame 0, Default {
                          }
                          frame 1 {
                            w470 = 0.0 ("AC Frequency (kHz)")
                          }
                        }
                        n77 = formula code="f100=f200 +c1 +(c2-c1)*(time/t1)**g1;\n\nV=f100;"("c1"=w445, "time"=w439, "t1"=w449, "c2"=w444, "f200"=w443, "fmod"=w448, "A1"=w447, "A2"=w446, "g1"=w440, "g2"=w442) -> ("f100"=w434:dbl, "time"=w435:dbl, "V"=w431:dbl)
                        n78 = Divide(x=w438, y=w437) -> (x/y=w436:dbl)
                      }
                    }
                  }
                  n79 = Add(x=w127, y=w125) -> (x+y=w123:dbl[])
                  n80 = Build Array (concatenate)(w122, w123) -> (w128:dbl[])
                  n81 = Build Array (concatenate)(w119, w120) -> (w121:dbl[])
                }
              }
            }
          }
        }
        n82 = case shown="True" w69 {
          tunnel: [0.0 w83] -> w70
          tunnel: w71 -> [_ w83]
          frame False {
          }
          frame True {
          }
        }
        n83 = Build Array (concatenate)(w72, w70) -> (w64:dbl[])
        n84 = Bundle By Name("dt"=w66, "Y"=w64) -> (w68:waveform(dbl))  [unwired: 1 in]
      }
      "Voltage\nArrays" <- w6
      "signal out" <- w11
      n85 = Array Size(array=w9) -> (size(s)=w8:i32)
      n86 = Index Array(array=w6, index (row)=0, index (col)=100 ("disabled index (col)")) -> (element=→"redMOTAOMVoltage":dbl)
    }
    frame #1 {
      w477 = T3 3 items=["no dialog", "OK message", "continue or stop message", "OK message + warnings", "continue/stop + warnings"] ("type of dialog (OK msg:1)")
      w478 = 10123 items=["Finite Samples"=10178, "Continuous Samples"=10123, "Hardware Timed Single Point"=12522] ("sample mode")
      w479 = 10280 items=["Rising"=10280, "Falling"=10171] ("edge")
      w489 = 10214 items=["High"=10192, "Low"=10214] ("idle state")
      w490 = 10178 items=["Finite Samples"=10178, "Continuous Samples"=10123, "Hardware Timed Single Point"=12522] ("sample mode")
      # "Counter Channel"
      # "Physical Channel"
      # "device 9:\n6733 board"
      # "task ID is an output of this VI; it is used to close the 6733 later in the program.\nDo not delete!"
      # "sampling rate"
      # "total points per channel"
      # "Points per segment"
      # "write voltage values to intermediate buffer"
      # "write waveform"
      # "Configure counter\nfor retriggerable AO"
      n87 = case shown="8" w523 {
        tunnel: [_ refnum<k21> "6733 AO 00" ("global virtual channels") refnum<k21> "6733 AO 00:01" ("global virtual channels") refnum<k21> "6733 AO 00:02" ("global virtual channels") refnum<k21> "6733 AO 00:03" ("global virtual channels") refnum<k21> "6733 AO 00:04" ("global virtual channels") refnum<k21> "6733 AO 00:05" ("global virtual channels") refnum<k21> "6733 AO 00:06" ("global virtual channels") refnum<k21> "6733 AO 00:07" ("global virtual channels")] -> w484
        frame 0, Default {
          n88 = call "Display Message to User2"() -> ("Cancel"=w538:bool)  [unwired: 10 in, 1 out]
          n89 = Stop(stop? (T)=w538) -> ()
        }
        frame 1 {
        }
        frame 2 {
        }
        frame 3 {
        }
        frame 4 {
        }
        frame 5 {
        }
        frame 6 {
        }
        frame 7 {
        }
        frame 8 {
        }
      }
      n90 = property class="DAQmx Device"("Active Device"=tag "Dev9") -> ("Identification:Product Type"=w518:string)  [unwired: 2 in, 2 out]
      n91 = Equal?(x=w518, y="PCI-6733") -> (x = y?=w521:bool)
      n92 = case shown="True" w521 {
        tunnel: [w534 "PCI-6733 OK"] -> w520
        tunnel: "error in" -> [w535 w536]
        tunnel: [w533 w536] -> w516
        frame False {
          w534 = "PCI-6221 not found."
          n93 = Unbundle(w535) -> ()  [unwired: 3 out]
          n94 = Bundle(cluster=w535, "source"=w534) -> (w533:errorcluster)  [unwired: 2 in]
        }
        frame True {
        }
      }
      "6733 Status" <- w520
      n95 = case shown="True" "Case Constant\n(See Context Help) 2" {
        tunnel: w513 -> [_ w527]
        tunnel: w514 -> [_ w526]
        tunnel: w516 -> [w524 w525]
        tunnel: [w524 w525] -> w485
        frame False {
        }
        frame True {
          # "Clears tasks _before_ writing new waveform.\nError is not hooked up so that program will finish\nrunning either way."
          n96 = call <vilib>:"DAQmx Stop Task.vi"("task/channels in"=w526) -> ("task out"=w531:refnum<k21>, "error out"=w532:errorcluster)  [unwired: 13 in]
          n97 = call <vilib>:"DAQmx Clear Task.vi"("task in"=w531, "error in"=w532) -> ("error out"=w528:errorcluster)  [unwired: 13 in]
          n98 = call <vilib>:"DAQmx Stop Task.vi"("task/channels in"=w527, "error in"=w528) -> ("task out"=w529:refnum<k21>, "error out"=w530:errorcluster)  [unwired: 12 in]
          n99 = call <vilib>:"DAQmx Clear Task.vi"("task in"=w529, "error in"=w530) -> ()  [unwired: 13 in, 1 out]
        }
      }
      n100 = call <vilib>:"DAQmx Create Task.vi"("new task name"="Red Waveform", "auto cleanup"=FALSE, "global virtual channels"=w484, "error in"=w485) -> ("task out"=w512:refnum<k21>, "error out"=w508:errorcluster)  [unwired: 10 in]
      n101 = call-poly <vilib>:"DAQmx Timing.vi"("task/channels in"=w512, "sample mode"=w478, "rate"=w476, "source"=tag "/Dev9/Ctr0InternalOutput", "error in"=w508) -> ("task out"=w511:refnum<k21>, "error out"=w507:errorcluster)  [unwired: 9 in]
      n102 = call-poly <vilib>:"DAQmx Write.vi"("task/channels in"=w511, "data"=w475, "timeout"=10.0, "error in"=w507) -> ("task out"=w510:refnum<k21>, "error out"=w486:errorcluster)  [unwired: 9 in, 1 out]
      n103 = call <vilib>:"DAQmx Create Task.vi"("new task name"="6733 Counter Output", "auto cleanup"=FALSE, "error in"=w486) -> ("task out"=w499:refnum<k21>, "error out"=w498:errorcluster)  [unwired: 11 in]
      n104 = call-poly <vilib>:"DAQmx Create Virtual Channel.vi"("task in"=w499, "frequency"=w476, "counter"=tag "Dev9/ctr0", "error in"=w498, "idle state"=w489) -> ("task out"=w500:refnum<k21>, "error out"=w497:errorcluster)  [unwired: 9 in]
      n105 = call-poly <vilib>:"DAQmx Timing.vi"("task/channels in"=w500, "sample mode"=w490, "samples per channel"=w474, "error in"=w497) -> ("task out"=w501:refnum<k21>, "error out"=w496:errorcluster)  [unwired: 10 in]
      n106 = call-poly <vilib>:"DAQmx Trigger.vi"("task/channels in"=w501, "source"=tag "/Dev9/PFI6", "edge"=w479, "error in"=w496) -> ("task out"=w502:refnum<k21>, "error out"=w495:errorcluster)  [unwired: 10 in]
      n107 = property class="DAQmx Trigger"(reference=w502, error in=w495, "Start:More:Retriggerable"=TRUE) -> (reference out=w503:refnum<k21>, error out=w494:errorcluster)
      n108 = call <vilib>:"DAQmx Start Task.vi"("task/channels in"=w510, "error in"=w494) -> ("task out"=→"6733 adiabatic loading task out":refnum<k21>, "error out"=w493:errorcluster)  [unwired: 12 in]
      n109 = call <vilib>:"DAQmx Start Task.vi"("task/channels in"=w503, "error in"=w493) -> ("task out"=→"6733 counter task out":refnum<k21>, "error out"=→"error out":errorcluster)  [unwired: 12 in]
      n110 = call <vilib>:"Simple Error Handler.vi"("type of dialog (OK msg:1)"=w477) -> ()  [unwired: 4 in, 5 out]
      "wvfrm size" <- w474
    }
  }
